vi "Measure Output.vi"(8 "error in":errorcluster, 11 "3300 in":refnum<class "3300.lvclass">) -> (0 "error out":errorcluster, 1 "Current":dbl[](array[numeric]), 2 "Voltage":dbl[](array[numeric]), 3 "3300 out":refnum<class "3300.lvclass">)   [LabVIEW 2019, in "3300.lvlib" / "3300.lvclass"]
uses:
  Library/3300.lvclass
  C:/Users/Public/Documents/Development/builds/Instruments/Electronic Load.lvlibp/Library/Electronic Load.lvclass
  builds/Instruments/Electronic Load.lvlibp/Accessors/Read Available Channels.vi
  builds/Instruments/Electronic Load.lvlibp/Accessors/Status/Write Status_Flags.vi
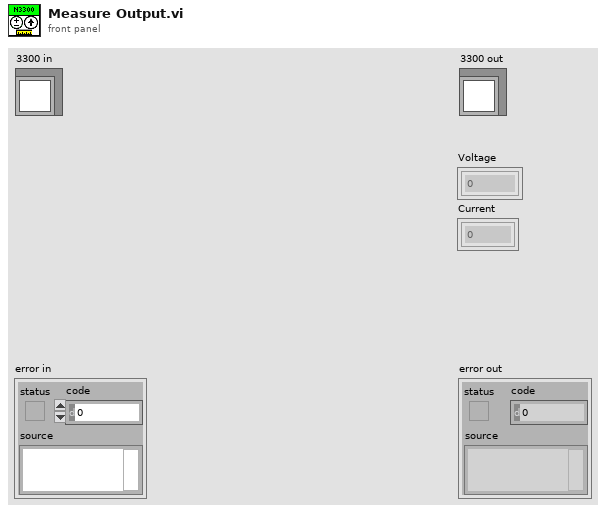
[diagram p1: front panel]
types:
  T1 = typedef "Electronic Load.lvlibp/Electronic Load.lvclass/Status_Flags.ctl" = cluster{"Interlock":bool, "OVP":bool, "OCP":bool, "Output":bool}
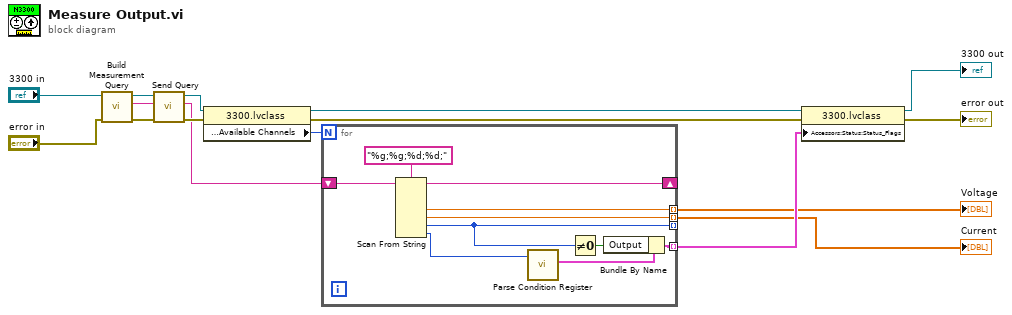
[diagram p0: block diagram]
diagram:
  n1 = call "Build Measurement Query.vi"("error in"="error in", "3300 in"="3300 in") -> ("error out"=w14:errorcluster, "Measurement Query"=w12:string, "3300 out"=w13:refnum<class "3300.lvclass">)  [unwired: 7 in]
  n2 = call "Send Query.vi"("error in"=w14, "Query"=w12, "3300 in"=w13) -> ("error out"=w10:errorcluster, "Read Data"=w1:string, "3300 out"=w11:refnum<class "3300.lvclass">)  [unwired: 6 in]
  n3 = property class="3300.lvclass"(reference=w11, error in=w10) -> (reference out=w8:refnum<class "3300.lvclass">, error out=w9:errorcluster, "Accessors:Configuration:Available Channels"=w2:i32)
  n4 = for {
    N: w2 -> [_]
    tunnel: [w24] -> w5 mode=indexing
    shift-right: [w22] -> _
    shift-left: w1 -> [w23]
    tunnel: [w20] -> w4 mode=indexing
    tunnel: [w19] -> w3 mode=indexing
    tunnel: [w17] -> _ mode=indexing
    n5 = Scan From String(format string="%g;%g;%d;%d;", input string=w23) -> (remaining string=w22:string, output 1=w20:dbl, output 2=w19:dbl, output 3=w17:i32, output 4=w18:i32)  [unwired: 6 in, 2 out]
    n6 = call "Parse Condition Register.vi"("Condition_Register"=w18) -> ("Status_Flags"=w26:T1)  [unwired: 10 in]
    n7 = Not Equal To 0?(x=w17) -> (x != 0?=w25:bool)
    n8 = Bundle By Name(cluster=w26, "Output"=w25) -> (w24:T1)
  }
  "Voltage" <- w4
  "Current" <- w3
  n9 = property class="3300.lvclass"(reference=w8, error in=w9, "Accessors:Status:Status_Flags"=w5) -> (reference out=→"3300 out":refnum<class "3300.lvclass">, error out=→"error out":errorcluster)
